vi "algorithm5.vi"(10 "String":string) -> (2 "y":i32)   [LabVIEW 2017]
panel:
  out "Array":i32[][](array[numeric])
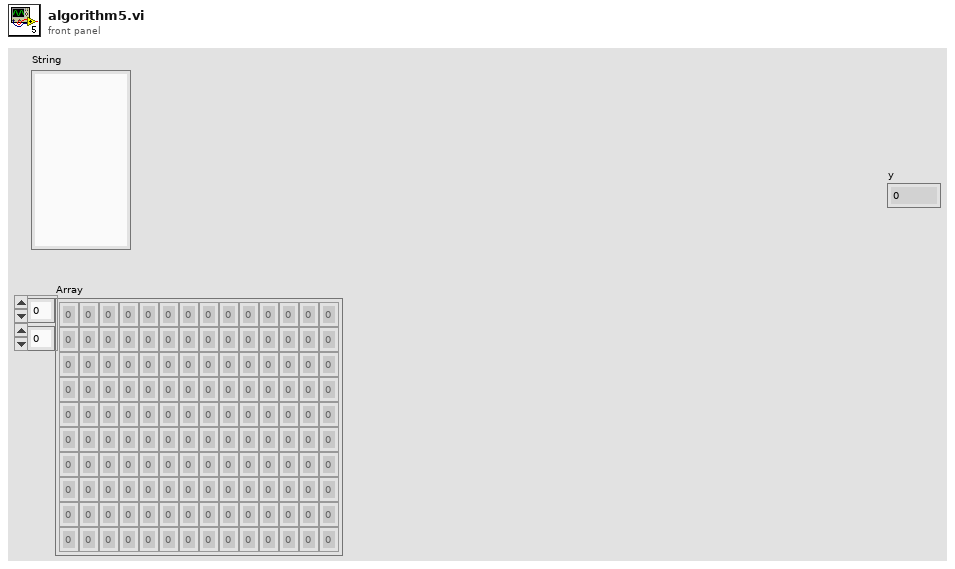
[diagram p1: front panel]
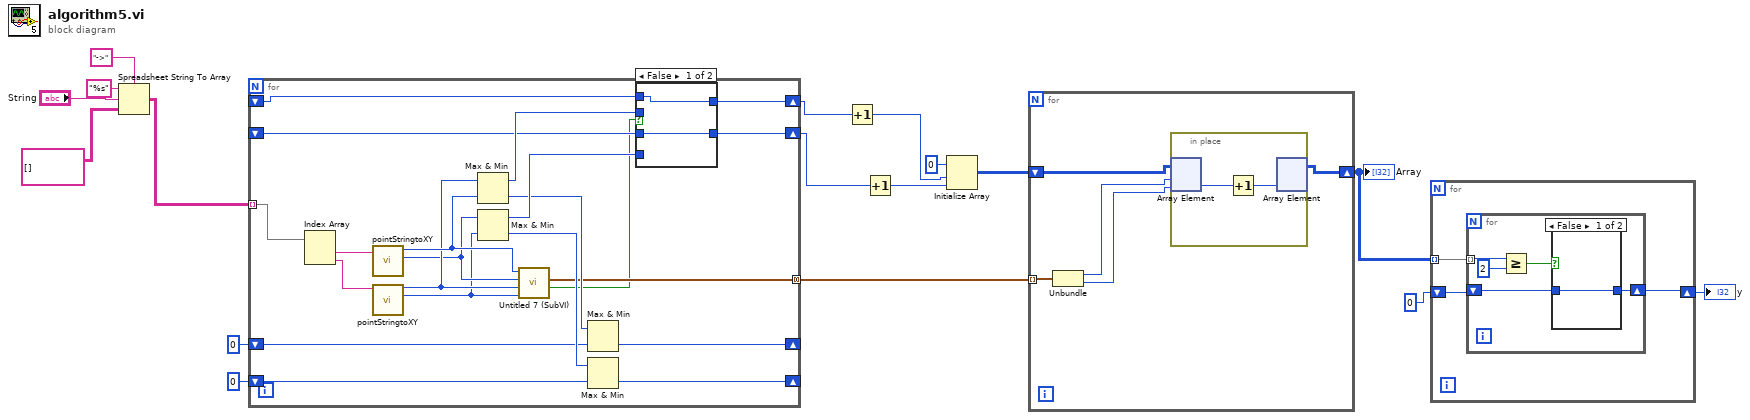
[diagram p0: block diagram]
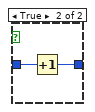
[diagram p2: hidden frame]
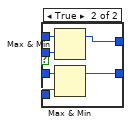
[diagram p3: hidden frame]
diagram:
  n1 = Spreadsheet String To Array(delimiter (Tab)="->", format string="%s", spreadsheet string="String", array type (2D Dbl)=string[][] []) -> (array=w13:string[][])
  n2 = for {
    tunnel: w13 -> [w38] mode=indexing
    shift-right: [w27] -> _
    shift-left: 0 -> [w26]
    shift-right: [w25] -> _
    shift-left: 0 -> [w24]
    shift-right: [w23] -> w9
    shift-left: _ -> [w22]
    shift-right: [w21] -> w8
    shift-left: _ -> [w20]
    tunnel: [w19] -> w7 mode=concatenating
    n3 = Index Array(array=w38) -> (element #1=w37:string, element #2=w36:string)  [unwired: 2 in]
    n4 = call "pointStringtoXY.vi"("stringPoint"=w37) -> ("y"=w33:i32, "x"=w35:i32)  [unwired: 9 in]
    n5 = call "pointStringtoXY.vi"("stringPoint"=w36) -> ("y"=w32:i32, "x"=w34:i32)  [unwired: 9 in]
    n6 = Max & Min(x=w34, y=w35) -> (max(x,y)=w31:i32, min(x,y)=w29:i32)
    n7 = Max & Min(x=w33, y=w32) -> (max(x,y)=w30:i32, min(x,y)=w28:i32)
    n8 = call "Untitled 7 (SubVI).vi"("y 2"=w32, "x 2"=w34, "y 1"=w33, "x 1"=w35) -> ("Boolean"=w18:bool, "Array"=w19:cluster{"x 1":i32, i32}[])  [unwired: 6 in]
    n9 = Max & Min(x=w29, y=w26) -> (min(x,y)=w27:i32)  [unwired: 1 out]
    n10 = Max & Min(x=w28, y=w24) -> (min(x,y)=w25:i32)  [unwired: 1 out]
    n11 = case shown="False" w18 {
      tunnel: w31 -> [_ w46]
      tunnel: w30 -> [_ w45]
      tunnel: [w40 w44] -> w23
      tunnel: w22 -> [w40 w43]
      tunnel: [w39 w42] -> w21
      tunnel: w20 -> [w39 w41]
      frame False {
      }
      frame True {
        n12 = Max & Min(x=w43, y=w46) -> (max(x,y)=w44:i32)  [unwired: 1 out]
        n13 = Max & Min(x=w41, y=w45) -> (max(x,y)=w42:i32)  [unwired: 1 out]
      }
    }
  }
  n14 = Increment(x=w9) -> (x+1=w2:i32)
  n15 = Increment(x=w8) -> (x+1=w1:i32)
  n16 = Initialize Array(0 ("element"), w2, w1) -> (w6:i32[][])
  n17 = for {
    tunnel: w7 -> [w51] mode=indexing
    shift-right: [w47] -> w5
    shift-left: w6 -> [w50]
    n18 = Unbundle(w51) -> ("x 1"=w49:i32, w48:i32)
    n19 = in-place {
      n20 = in-place-array #1(w50, w49, w48) -> (w53:i32)
      n21 = Increment(x=w53) -> (x+1=w52:i32)
      n22 = in-place-array #1(w52) -> (w47:i32[][])  [unwired: 2 out]
    }
  }
  "Array" <- w5
  n23 = for {
    tunnel: w5 -> [w56] mode=indexing
    shift-right: [w55] -> w3
    shift-left: 0 ("y") -> [w54]
    n24 = for {
      tunnel: w56 -> [w61] mode=indexing
      shift-right: [w58] -> w55
      shift-left: w54 -> [w57]
      n25 = Greater Or Equal?(x=w61, y=2) -> (x >= y?=w59:bool)
      n26 = case shown="False" w59 {
        tunnel: [w62 w64] -> w58
        tunnel: w57 -> [w62 w63]
        frame False {
        }
        frame True {
          n27 = Increment(x=w63) -> (x+1=w64:i32)
        }
      }
    }
  }
  "y" <- w3
